vi "MB_Slaver.vi"() -> ()   [LabVIEW 2015]
doc: "Modbus主机模式"
uses:
  lib/pcomm/PCOMM.lvlib
panel:
  in  "接收帧":string caption="Rx Frame"
  in  "发送帧":string caption="Tx Frame"
  in  "Input Num":u8=1 min=1 format="%02x"
  in  "Input Addr":u16 caption="Addr" format="%04x"
  in  "Coil Num":u8=1 min=1 format="%02x"
  in  "Coil Addr":u16 format="%04x"
  in  "Holding Reg Num":u8 format="%02x"
  in  "Holding Reg Addr":u16 caption="Addr" format="%04x"
  in  "Input Reg Num":u8 format="%02x"
  in  "Input Reg Addr":u16 caption="Addr" format="%04x"
  in  "从机编号":u8 format="%02x"
  in  "Holding Register":u16[](array[numeric]) format="%04x"
  in  "Input Register":u16[](array[numeric]) format="%04x"
  in  "Input":bool[][](array[boolean])=[[FALSE, FALSE, FALSE, FALSE, FALSE, FALSE, FALSE, FALSE]]
  in  "Coils":bool[][](array[boolean])=[[FALSE, FALSE, FALSE, FALSE, FALSE, FALSE, FALSE, FALSE]]
  in  "刷新按钮":bool
  in  "字符串":string="串口设置"
  in  "串口号":i32(ring)=1 items=["COM1 通信端口 (COM1)"=1, "COM2 ELTIMA Virtual Serial Port (COM2->COM3)"=2, "COM3 ELTIMA Virtual Serial Port (COM3->COM2)"=3, "COM8 USB-SERIAL CH340 (COM8)"=8]
  in  "奇偶校验":i32(ring)=8 caption="校   验" items=["None"=0, "Odd"=8, "Even"=24, "Mark"=40, "Space"=56]
  in  "数据比特":i32(ring)=3 caption="数据位" items=["5", "6", "7", "8"]
  in  "波特率":i32(ring)=16 items=["1800"=8, "2400"=9, "4800"=10, "7200"=11, "9600"=12, "19200"=13, "38400"=14, "57600"=15, "115200"=16, "230400"=17, "460800"=18, "921600"=19]
  in  "停止位":i32(ring) items=["1"=0, "2"=4]
  in  "打开/关闭串口":bool
  in  "Rx":u32
  in  "Tx":u32
  in  "通信模式":enum16{"RTU", "ASCII"}(ring)
  in  "主从选择":enum32{"Slaver"}(ring)
  in  "接收帧分析":string
  # "RTU模式不会去检测字符间超时事件"
  # "主从模式"
  # "通信模式"
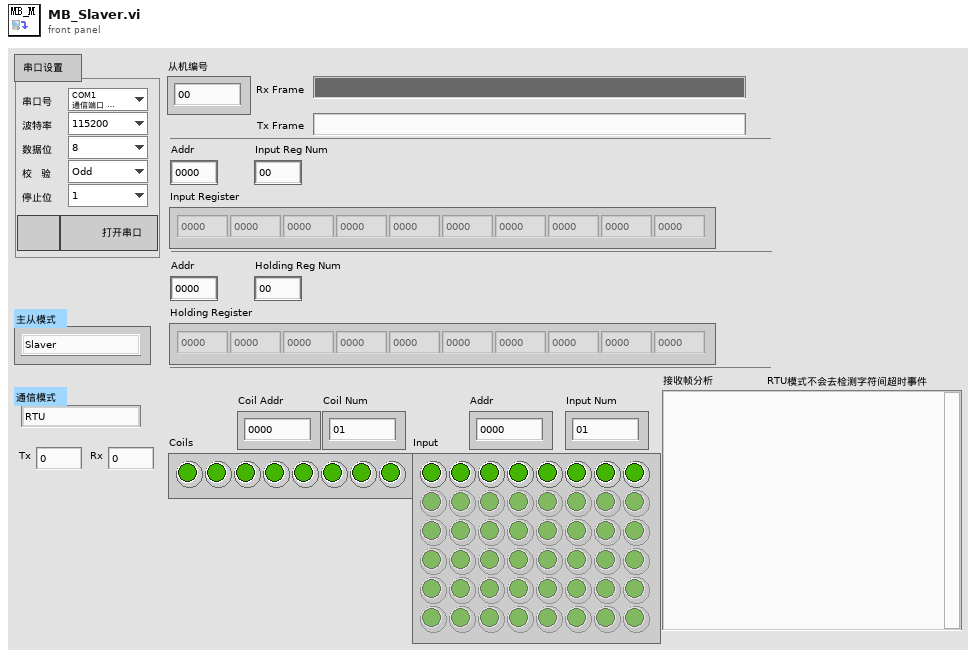
[diagram p1: front panel]
types:
  T1 = enum8{"Enabled", "Disabled", "Disabled and Grayed Out"}
  T2 = typedef "LVPointTypeDef.ctl" = cluster{"Horizontal":i16, "Vertical":i16}
  T3 = typedef "LVRectTypeDef.ctl" = cluster{"Left":i16, "Top":i16, "Right":i16, "Bottom":i16}
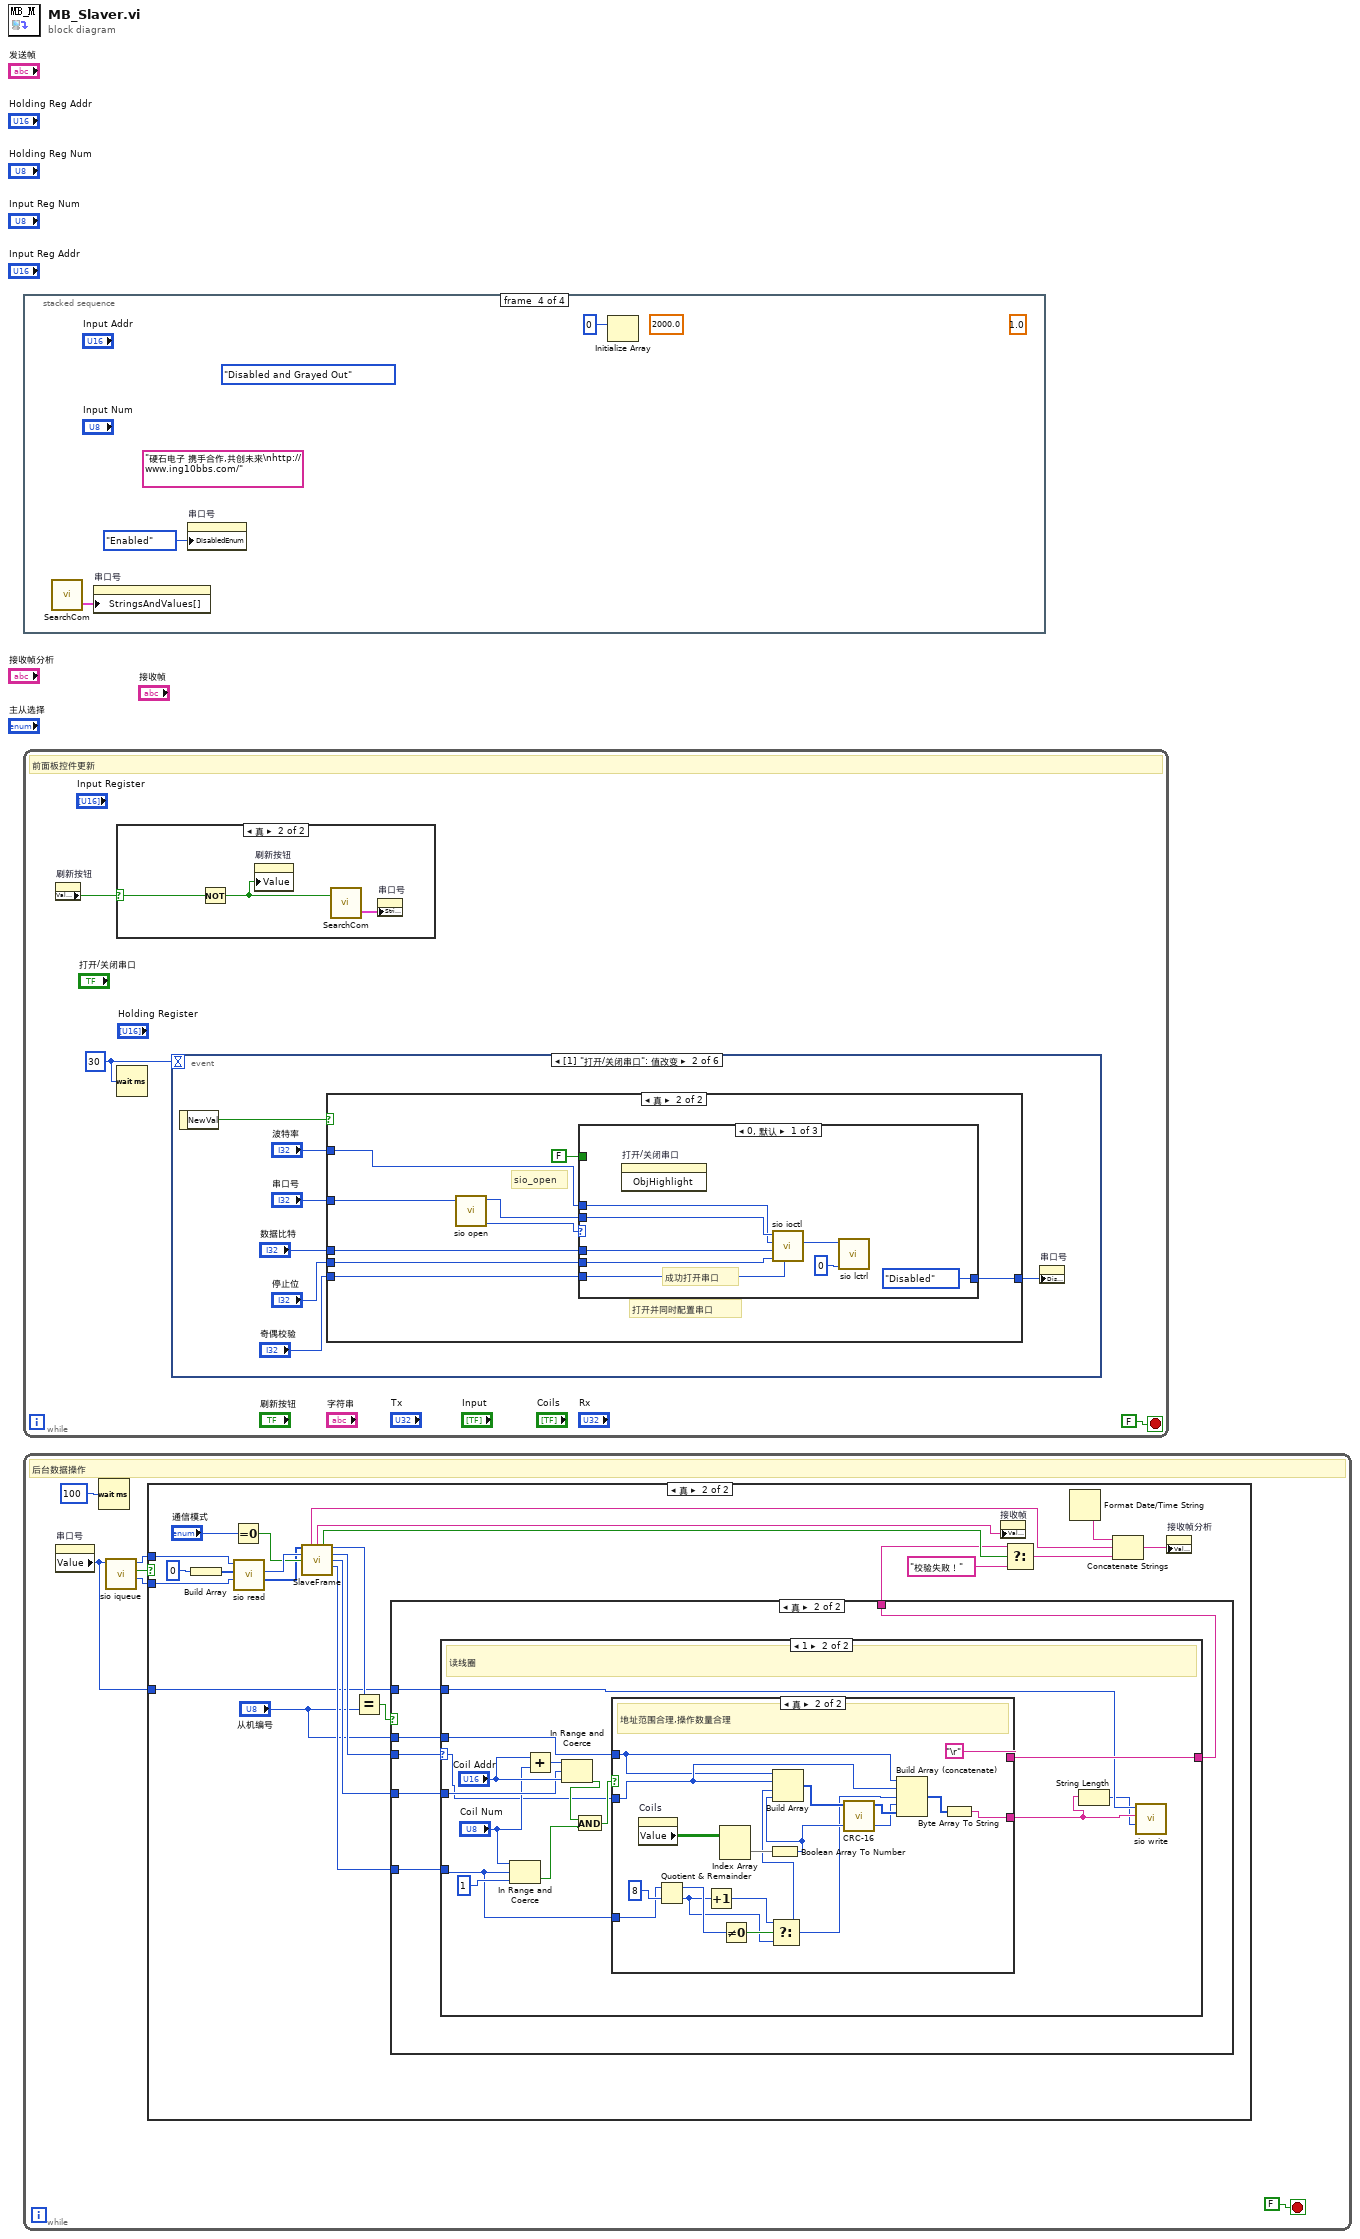
[diagram p0: block diagram]
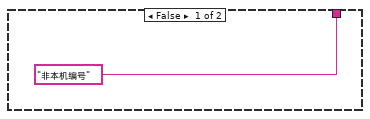
[diagram p3: hidden frame]
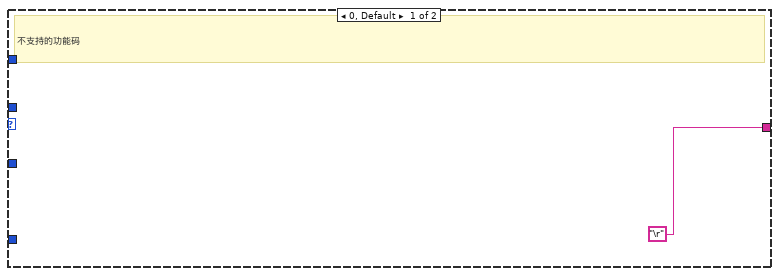
[diagram p4: hidden frame]
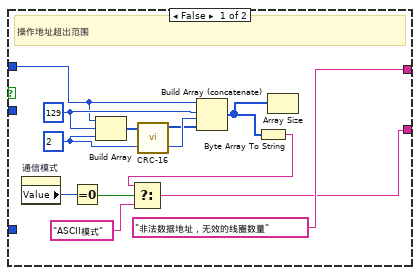
[diagram p5: hidden frame]
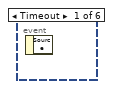
[diagram p6: hidden frame]
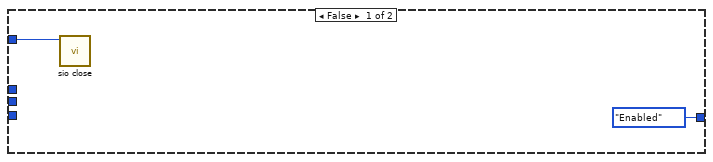
[diagram p7: hidden frame]
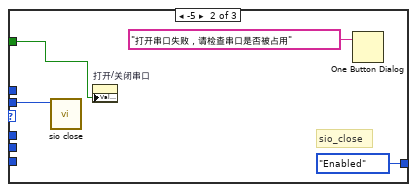
[diagram p8: hidden frame]
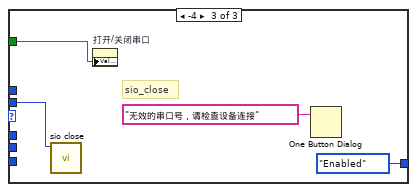
[diagram p9: hidden frame]
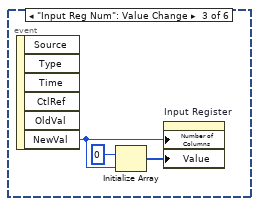
[diagram p10: hidden frame]
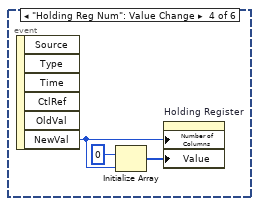
[diagram p11: hidden frame]
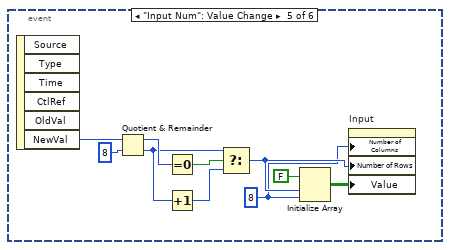
[diagram p12: hidden frame]
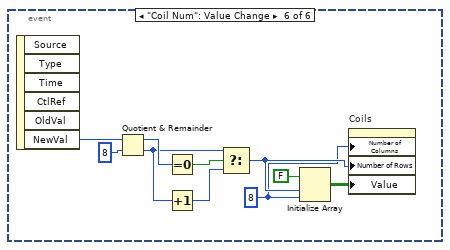
[diagram p13: hidden frame]
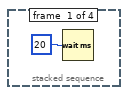
[diagram p15: hidden frame]
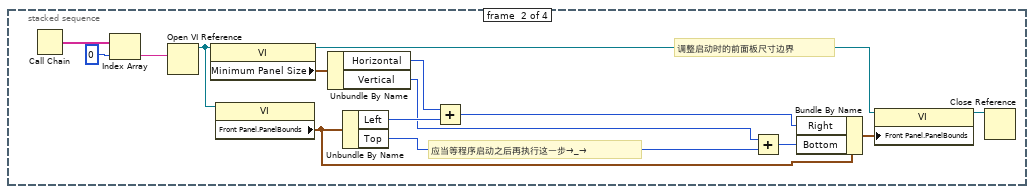
[diagram p16: hidden frame]
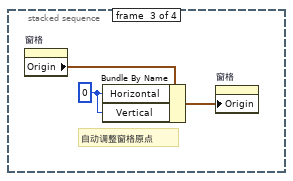
[diagram p17: hidden frame]
diagram:
  n1 = stacked-sequence {
    frame #0 {
      n2 = Wait (ms)(milliseconds to wait=u32 20) -> ()  [unwired: 1 out]
    }
    frame #1 {
      # "调整启动时的前面板尺寸边界"
      # "应当等程序启动之后再执行这一步→_→"
      n3 = Call Chain ("调用链")() -> (call chain=w4:string[])
      n4 = Index Array(array=w4, index=0) -> (element=w2:string)
      n5 = Open VI Reference(vi path=w2) -> (vi reference=w14:refnum<vi>)  [unwired: 1 in, 5 out]
      n6 = property class="VI"(reference=w14) -> (reference out=w15:refnum<vi>, "Minimum Panel Size"=w5:T2)  [unwired: 1 in, 1 out]
      n7 = property class="VI"(reference=w14) -> ("Front Panel.PanelBounds"=w11:T3)  [unwired: 1 in, 2 out]
      n8 = Unbundle By Name(w5) -> ("Horizontal"=w12:i16, "Vertical"=w9:i16)
      n9 = Unbundle By Name(w11) -> ("Left"=w13:i16, "Top"=w8:i16)
      n10 = Add(x=w12, y=w13) -> (x+y=w10:i16)
      n11 = Add(x=w9, y=w8) -> (x+y=w7:i16)
      n12 = Bundle By Name(cluster=w11, "Right"=w10, "Bottom"=w7) -> (w6:T3)
      n13 = property class="VI"(reference=w15, "Front Panel.PanelBounds"=w6) -> (reference out=w16:refnum<vi>)  [unwired: 1 in, 1 out]
      n14 = Close Reference(reference=w16) -> ()  [unwired: 1 in, 1 out]
    }
    frame #2 {
      w19 = i16 0
      # "自动调整窗格原点"
      n15 = property on="窗格" class="Pane"() -> ("Origin"=w18:T2)  [unwired: 2 in, 2 out]
      n16 = Bundle By Name(cluster=w18, "Horizontal"=w19, "Vertical"=w19) -> (w17:T2)
      n17 = property on="窗格" class="Pane"("Origin"=w17) -> ()  [unwired: 2 in, 2 out]
    }
    frame #3 {
      (unwired) T1."Disabled and Grayed Out" ("禁用")
      (unwired) 1.0
      (unwired) 2000.0
      (unwired) "硬石电子 携手合作,共创未来\nhttp://www.ing10bbs.com/"
      n18 = call "SearchCom.vi"() -> ("下拉列表项"=w22:cluster{"String":string, "Value":i32}[])  [unwired: 3 in]
      n19 = property on="串口号" class="Ring (严格)"("StringsAndValues[]"=w22) -> ()  [unwired: 2 in, 2 out]
      n20 = property on="串口号" class="Ring (严格)"("DisabledEnum"=T1."Enabled" ("禁用")) -> ()  [unwired: 2 in, 2 out]
      n21 = Initialize Array(u8 0 ("值")) -> ()  [unwired: 1 in, 1 out]
    }
  }
  n22 = while {
    stop <- FALSE stop-if-true
    w23 = 30
    # "前面板控件更新"
    n23 = property on="刷新按钮" class="Bool (严格)"() -> ("Value"=w24:bool)  [unwired: 2 in, 2 out]
    n24 = case shown="真" w24 {
      selector: w24 -> [_ w87]
      frame False {
      }
      frame True {
        n25 = Not(x=w87) -> (.not. x?=w86:bool)
        n26 = property on="刷新按钮" class="Bool (严格)"("Value"=w86) -> ()  [unwired: 2 in, 2 out]
        n27 = call "SearchCom.vi"("使用注册表？"=w86) -> ("下拉列表项"=w88:cluster{"String":string, "Value":i32}[])  [unwired: 2 in]
        n28 = property on="串口号" class="Ring (严格)"("StringsAndValues[]"=w88) -> ()  [unwired: 2 in, 2 out]
      }
    }
    n29 = Wait (ms)(milliseconds to wait=w23) -> ()  [unwired: 1 out]
    n30 = event shown="[1] \"打开/关闭串口\": 值改变" {
      selector: _ -> [_ _ _ _ _ _]
      dyn-events: _ -> [_ _ _ _ _ _]
      timeout: w23 -> [_ _ _ _ _ _]
      event Timeout {
        n31 = event-data() -> ()  [unwired: 1 in, 1 out]
      }
      event "打开/关闭串口": Value Change {
        n32 = event-data() -> ("NewVal"=w31:bool)  [unwired: 1 in]
        n33 = case shown="真" w31 {
          tunnel: [T1."Enabled" w43] -> w32
          tunnel: "串口号" -> [w33 w42]
          tunnel: "奇偶校验" -> [_ w38]
          tunnel: "停止位" -> [_ w37]
          tunnel: "数据比特" -> [_ w36]
          tunnel: "波特率" -> [_ w35]
          frame False {
            n34 = call "sio close.vi"("port"=w33) -> ()  [unwired: 9 in, 2 out]
          }
          frame True {
            # "sio_open"
            # "打开并同时配置串口"
            n35 = call "sio open.vi"("port"=w42) -> ("port"=w41:i32, "Status"=w40:i32)  [unwired: 6 in]
            n36 = case shown="0, 默认" w40 {
              tunnel: w41 -> [w50 w53 w57]
              tunnel: [T1."Disabled" T1."Enabled" T1."Enabled"] -> w43
              tunnel: FALSE -> [_ w52 w56]
              tunnel: w38 -> [w49 _ _]
              tunnel: w37 -> [w48 _ _]
              tunnel: w36 -> [w47 _ _]
              tunnel: w35 -> [w46 _ _]
              frame 0, Default {
                # "成功打开串口"
                n37 = invoke on="打开/关闭串口" class="Bool (严格)" method="ObjHighlight"() -> ()  [unwired: 3 in, 3 out]
                n38 = call "sio ioctl.vi"("parity"=w49, "stop bits"=w48, "data bits"=w47, "baud"=w46, "port"=w50) -> ("port"=w45:i32)  [unwired: 5 in, 1 out]
                n39 = call "sio lctrl.vi"("mode"=0, "port"=w45) -> ()  [unwired: 8 in, 2 out]
              }
              frame -5 {
                # "sio_close"
                n40 = call "sio close.vi"("port"=w53) -> ()  [unwired: 9 in, 2 out]
                n41 = property on="打开/关闭串口" class="Bool (严格)"("Value"=w52) -> ()  [unwired: 2 in, 2 out]
                n42 = One Button Dialog(message="打开串口失败，请检查串口是否被占用") -> ()  [unwired: 1 in, 1 out]
              }
              frame -4 {
                # "sio_close"
                n43 = call "sio close.vi"("port"=w57) -> ()  [unwired: 9 in, 2 out]
                n44 = property on="打开/关闭串口" class="Bool (严格)"("Value"=w56) -> ()  [unwired: 2 in, 2 out]
                n45 = One Button Dialog(message="无效的串口号，请检查设备连接") -> ()  [unwired: 1 in, 1 out]
              }
            }
          }
        }
        n46 = property on="串口号" class="Ring (严格)"("DisabledEnum"=w32) -> ()  [unwired: 2 in, 2 out]
      }
      event "Input Reg Num": Value Change {
        n47 = event-data() -> ("NewVal"=w61:u8)  [unwired: 1 in, 5 out]
        n48 = Initialize Array(0, w61) -> (w62:i32[])
        n49 = property on="Input Register" class="Arr (严格)"("Number of Columns"=w61, "Value"=w62) -> ()  [unwired: 2 in, 2 out]
      }
      event "Holding Reg Num": Value Change {
        n50 = event-data() -> ("NewVal"=w64:u8)  [unwired: 1 in, 5 out]
        n51 = Initialize Array(0, w64) -> (w65:i32[])
        n52 = property on="Holding Register" class="Arr (严格)"("Number of Columns"=w64, "Value"=w65) -> ()  [unwired: 2 in, 2 out]
      }
      event "Input Num": Value Change {
        w66 = 8
        n53 = event-data() -> ("NewVal"=w75:u8)  [unwired: 1 in, 5 out]
        n54 = Quotient & Remainder(x=w75, y=8) -> (x-y*floor(x/y)=w73:i32, floor(x/y)=w71:i32)
        n55 = Equal To 0?(x=w73) -> (x = 0?=w72:bool)
        n56 = Increment(x=w71) -> (x+1=w70:i32)
        n57 = Select(t=w71, s=w72, f=w70) -> (s? t:f=w67:i32)
        n58 = Initialize Array(FALSE, w67, w66) -> (w68:bool[][])
        n59 = property on="Input" class="Arr (严格)"("Number of Columns"=w66, "Number of Rows"=w67, "Value"=w68) -> ()  [unwired: 2 in, 2 out]
      }
      event "Coil Num": Value Change {
        w76 = 8
        n60 = event-data() -> ("NewVal"=w85:u8)  [unwired: 1 in, 5 out]
        n61 = Quotient & Remainder(x=w85, y=8) -> (x-y*floor(x/y)=w83:i32, floor(x/y)=w81:i32)
        n62 = Equal To 0?(x=w83) -> (x = 0?=w82:bool)
        n63 = Increment(x=w81) -> (x+1=w80:i32)
        n64 = Select(t=w81, s=w82, f=w80) -> (s? t:f=w77:i32)
        n65 = Initialize Array(FALSE, w77, w76) -> (w78:bool[][])
        n66 = property on="Coils" class="Arr (严格)"("Number of Columns"=w76, "Number of Rows"=w77, "Value"=w78) -> ()  [unwired: 2 in, 2 out]
      }
    }
  }
  n67 = while {
    stop <- FALSE stop-if-true
    # "后台数据操作"
    n68 = property on="串口号" class="Ring (严格)"() -> ("Value"=w89:i32)  [unwired: 2 in, 2 out]
    n69 = Wait (ms)(milliseconds to wait=100) -> ()  [unwired: 1 out]
    n70 = call "sio iqueue.vi"("port"=w89) -> ("len"=w90:i32, "not empty"=w92:bool, "port"=w91:i32)  [unwired: 8 in]
    n71 = case shown="真" w92 {
      tunnel: w91 -> [_ w117]
      tunnel: w90 -> [_ w114]
      tunnel: w89 -> [_ w95]
      frame False {
      }
      frame True {
        n72 = Build Array(i8 0) -> (w115:i8[])
        n73 = Equal To 0?(x="通信模式") -> (x = 0?=w108:bool)
        n74 = call "sio read.vi"("len"=w114, "buf"=w115, "port"=w117) -> ("buf out"=w104:i8[], "Status"=w109:i32)  [unwired: 4 in, 2 out]
        n75 = call "SlaveFrame.vi"("buf"=w104, "数组大小"=w109, "Mode"=w108) -> ("数据帧分析"=w107:string, "接收显示"=w106:string, "校验成功"=w105:bool, "从机编号"=w103:u8, "功能码"=w100:u8, "起始地址"=w99:u16, "寄存器/线圈数量"=w97:u16)  [unwired: 4 in, 2 out]
        n76 = Equal?(x=w103, y="从机编号") -> (x = y?=w102:bool)
        n77 = case shown="真" w102 {
          tunnel: ["非本机编号" w121] -> w101
          tunnel: w100 -> [_ w124]
          tunnel: w99 -> [_ w123]
          tunnel: w97 -> [_ w122]
          tunnel: "从机编号" -> [_ w120]
          tunnel: w95 -> [_ w119]
          frame False {
          }
          frame True {
            n78 = case shown="1" w124 {
              selector: w124 -> [_ w130]
              tunnel: w123 -> [_ w138]
              tunnel: w122 -> [_ w126]
              tunnel: ["\r" w132] -> w121
              tunnel: w120 -> [_ w131]
              tunnel: w119 -> [_ w129]
              frame 0, Default {
                # "不支持的功能码"
              }
              frame 1 {
                # "读线圈"
                n79 = In Range and Coerce(upper limit="Coil Num", x=w126, lower limit=u16 1) -> (In Range?=w134:bool)  [unwired: 1 out]
                n80 = Add(x="Coil Addr", y="Coil Num") -> (x+y=w140:u16)
                n81 = In Range and Coerce(upper limit=w140, x=w138, lower limit="Coil Addr") -> (In Range?=w135:bool)  [unwired: 1 out]
                n82 = And(x=w135, y=w134) -> (x .and. y?=w133:bool)
                n83 = case shown="真" w133 {
                  tunnel: ["非法数据地址，无效的线圈数量" "\r"] -> w132
                  tunnel: w131 -> [w142 w165]
                  tunnel: w130 -> [_ w166]
                  tunnel: [w141 w162] -> w128
                  tunnel: w126 -> [_ w160]
                  frame False {
                    w150 = u8 2
                    w151 = u8 129
                    # "操作地址超出范围"
                    n84 = property on="通信模式" class="Enum (严格)"() -> ("Value"=w147:enum16{"RTU", "ASCII"})  [unwired: 2 in, 2 out]
                    n85 = Equal To 0?(x=w147) -> (x = 0?=w148:bool)
                    n86 = Build Array(w142, w151, w150) -> (w152:u8[])
                    n87 = call "CRC-16.vi"("Frame in"=w152) -> ("CRC-16"=w149:u8[])  [unwired: 6 in]
                    n88 = Build Array (concatenate)(w142, w151, w150, w149) -> (w145:u8[])
                    n89 = Byte Array To String(unsigned byte array=w145) -> (string=w146:string)
                    n90 = Select(t=w146, s=w148, f="ASCII模式") -> (s? t:f=w141:string)
                    n91 = Array Size(array=w145) -> ()  [unwired: 1 out]
                  }
                  frame True {
                    # "地址范围合理,操作数量合理"
                    n92 = property on="Coils" class="Arr (严格)"() -> ("Value"=w169:bool[][])  [unwired: 2 in, 2 out]
                    n93 = Quotient & Remainder(x=w160, y=8) -> (x-y*floor(x/y)=w157:i32, floor(x/y)=w154:i32)
                    n94 = Increment(x=w154) -> (x+1=w155:i32)
                    n95 = Index Array(array=w169) -> (element=w168:bool[])  [unwired: 2 in]
                    n96 = Not Equal To 0?(x=w157) -> (x != 0?=w156:bool)
                    n97 = Boolean Array To Number(Boolean array=w168) -> (number=w158:u32)
                    n98 = Select(t=w155, s=w156, f=w154) -> (s? t:f=w153:i32)
                    n99 = Build Array(w165, w166, w153, w158) -> (w167:u32[])
                    n100 = call "CRC-16.vi"("Frame in"=w167) -> ("CRC-16"=w159:u8[])  [unwired: 6 in]
                    n101 = Build Array (concatenate)(w165, w166, w153, w158, w159) -> (w163:u32[])
                    n102 = Byte Array To String(unsigned byte array=w163) -> (string=w162:string)
                  }
                }
                n103 = String Length(string=w128) -> (length=w127:i32)
                n104 = call "sio write.vi"("len"=w127, "buf"=w128, "port"=w129) -> ()  [unwired: 6 in, 3 out]
              }
            }
          }
        }
        n105 = property on="接收帧" class="Str"("Value"=w106) -> ()  [unwired: 2 in, 2 out]
        n106 = Select(t=w101, s=w105, f="校验失败！") -> (s? t:f=w110:string)
        n107 = Format Date/Time String() -> (date/time string=w98:string)  [unwired: 3 in]
        n108 = Concatenate Strings(w98, w107, w110) -> (w112:string)
        n109 = property on="接收帧分析" class="Str"("Value"=w112) -> ()  [unwired: 2 in, 2 out]
      }
    }
  }
